vi "gentec-M-Link.Write.vi"(0 "VISA resource (In)":refnum<visa-resource-name>, 2 "Data To Write":string, 5 "error in (no error)":errorcluster) -> (14 "VISA resource (Out)":refnum<visa-resource-name>, 16 "Bytes Written":u32, 19 "error out":errorcluster)   [LabVIEW 2014, in "gentec-M-Link - Driver.lvlib"]
doc: "This VI calls a VISA Write."
uses:
  gentec-M-Link - Driver.lvlib
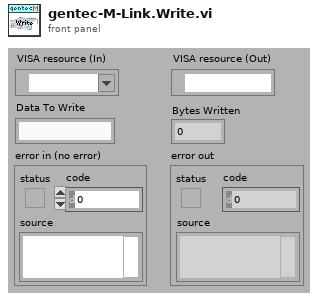
[diagram p1: front panel]
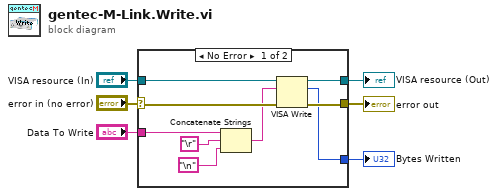
[diagram p0: block diagram]
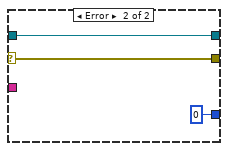
[diagram p2: hidden frame]
diagram:
  n1 = case shown="No Error" "error in (no error)" {
    selector: "error in (no error)" -> [w15 w18]
    tunnel: [w14 w18] -> w5
    tunnel: "VISA resource (In)" -> [w10 w17]
    tunnel: [w9 w17] -> w3
    tunnel: [w8 u32 0 ("return count")] -> w2
    tunnel: "Data To Write" -> [w7 _]
    frame No Error {
      n2 = Concatenate Strings(w7, "\r", "\n") -> (w12:string)
      n3 = VISA Write(VISA resource name=w10, write buffer=w12, error in (no error)=w15) -> (VISA resource name out=w9:refnum<visa-resource-name>, return count=w8:u32, error out=w14:errorcluster)
    }
    frame Error {
    }
  }
  "error out" <- w5
  "VISA resource (Out)" <- w3
  "Bytes Written" <- w2
